vi "PrefDialog.vi"(8 "error in (no error)":errorcluster, 11 "Agilent_3458":refnum<class "Agilent_3458.lvclass">) -> (0 "error out":errorcluster, 3 "Agilent_3458":refnum<class "Agilent_3458.lvclass">)   [LabVIEW 2018, in "DigitizerPlugins.lvlib" / "Agilent_3458.lvclass"]
uses:
  Agilent_3458.lvclass
  F:/Projects/ICDAS/NistPluggableModules/Digitizer/DigitizerPlugins/DigitizerBaseClass/DigitizerBase.lvclass
  F:/Program Files (x86)/National Instruments/LabVIEW 2018/user.lib/NIST/BaseClasses/BasePlugin_class/BasePlugin.lvclass
  DigitizerBaseClass/Typedefs/Channel.ctl
  DigitizerBaseClass/Typedefs/Trigger.ctl
  DigitizerBaseClass/Typedefs/TrigSource.ctl
  DigitizerBaseClass/Typedefs/Acquisition.ctl
  DigitizerBaseClass/DigitizerBase.lvclass/DigitizerBase.ctl
  Agilent_3458.lvclass/Agilent_3458.ctl
  <userlib>/NIST/BaseClasses/BasePlugin_class/BasePlugin.lvclass/BasePlugin.ctl
  DigitizerBaseClass/Accessors/Read Acquisition.vi
  Accessors/Read Function (0_ DC Voltage).vi
  DigitizerBaseClass/Accessors/Read Channels.vi
  DigitizerBaseClass/Accessors/Read Trigger.vi
  DigitizerBaseClass/Accessors/Read Handle.vi
  <userlib>/NIST/BaseClasses/BasePlugin_class/Accessors/Read PluginIniFilePath.vi
  DigitizerBaseClass/Accessors/Write Handle.vi
  DigitizerBaseClass/Accessors/Write Channels.vi
  DigitizerBaseClass/Accessors/Write Trigger.vi
  Accessors/Write Function (0_ DC Voltage).vi
  DigitizerBaseClass/Accessors/Write Acquisition.vi
  <userlib>/NIST/BaseClasses/BasePlugin_class/Accessors/Write PluginIniFilePath.vi
  <vilib>/Utility/config.llb/NI_LVConfig.lvlib
  DigitizerPlugins.lvlib
  DigitizerBaseClass/DigitizerBase.lvclass
panel:
  in  "Handle":string
  in  "btnSaveAs":bool
  in  "btnSave":bool
  in  "btnCancel":bool
  in  "Tab Control":enum32{"Channels", "Acquisition", "Trigger"}(tab)
  in  "Channel":T1
  in  "Function (0: DC Voltage)":u16(ring) items=["DC Voltage", "AC Voltage", "AC + DC Voltage", "DC Current", "AC Current", "AC + DC Current", "2-Wire Resistance", "4-Wire Resistance", "Frequency", "Period", "Direct Sampling DC", "Direct Sampling AC", "Sub-Sampling DC", "Sub-Sampling AC"]
  in  "Acquisition":T2 {"SampleMode" items=["Real Time", "Equivalent Time"]}
  in  "Trigger":T3
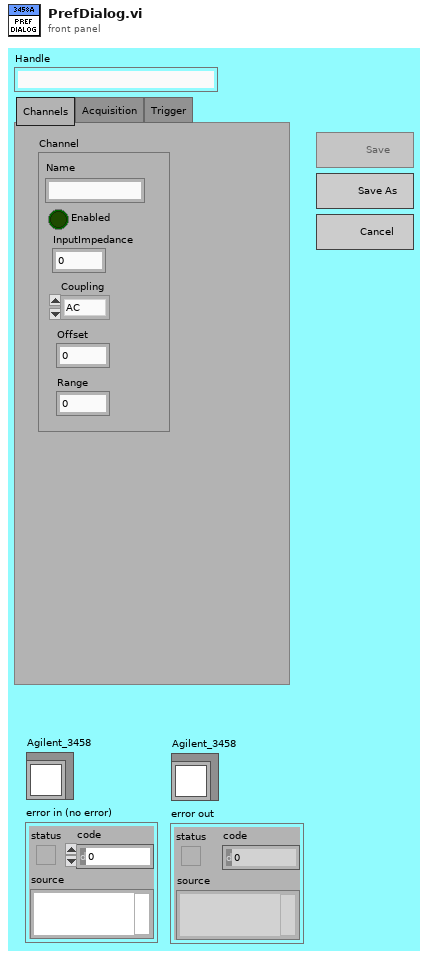
[diagram p1: front panel]
types:
  T1 = typedef "DigitizerPlugins.lvlib/DigitizerBase.lvclass/Channel.ctl" = cluster{"Name":string, "Enabled":bool, "InputImpedance":dbl, "Coupling":enum16{"AC", "DC", "Gnd"}, "Offset":dbl, "Range":dbl}
  T2 = typedef "DigitizerPlugins.lvlib/DigitizerBase.lvclass/Acquisition.ctl" = cluster{"SampleRate":dbl, "RecordSize":i32, "NumRecords":i32, "SampleMode":i32, "Timeout (ms)":i32}
  T3 = typedef "DigitizerPlugins.lvlib/DigitizerBase.lvclass/Trigger.ctl" = cluster{"Source":string, "Delay":dbl, "Holdoff":dbl, "PretriggerSamples":i32, "Sources":T4[]}
  T4 = typedef "DigitizerPlugins.lvlib/DigitizerBase.lvclass/TrigSource.ctl" = cluster{"Name":string, "Coupling":enum16{"AC", "DC", "HF Reject", "LF Reject", "Noise Reject"}, "Hysteresis":dbl, "Level":dbl, "Slope":enum16{"Positive", "Negative"}, "Type":enum16{"Edge", "Width", "Runt", "Glitch", "TV", "Window"}}
  T5 = enum32{"Invalid", "Default", "Floating", "Floating/Auto-Hide", "Modal"}
  T6 = enum8{"Enabled", "Disabled", "Disabled and Grayed Out"}
  T7 = typedef "NI_LVConfig.lvlib/Config Data RefNum.ctl" = refnum<k1>
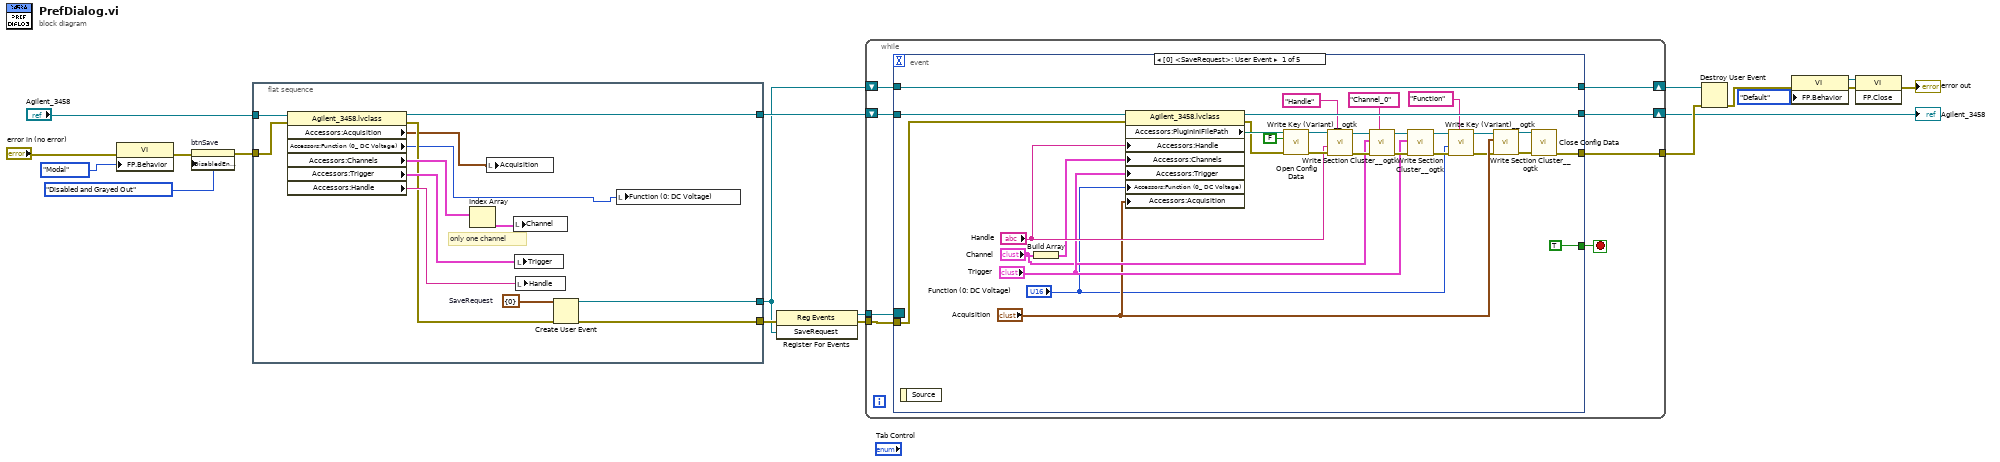
[diagram p0: block diagram]
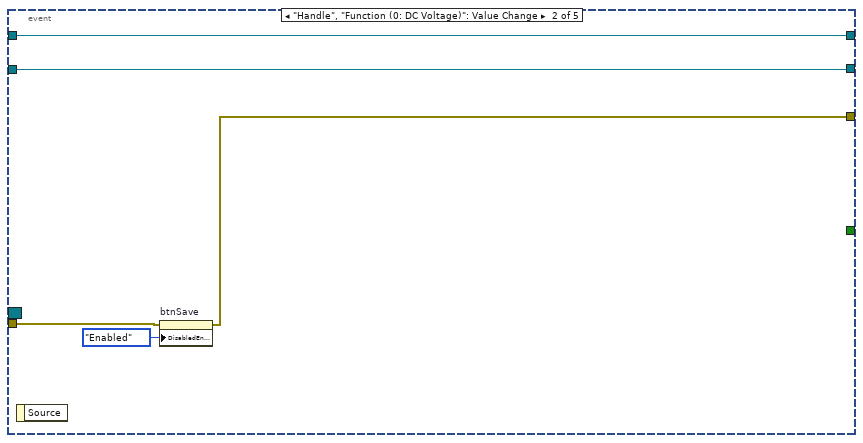
[diagram p2: hidden frame]
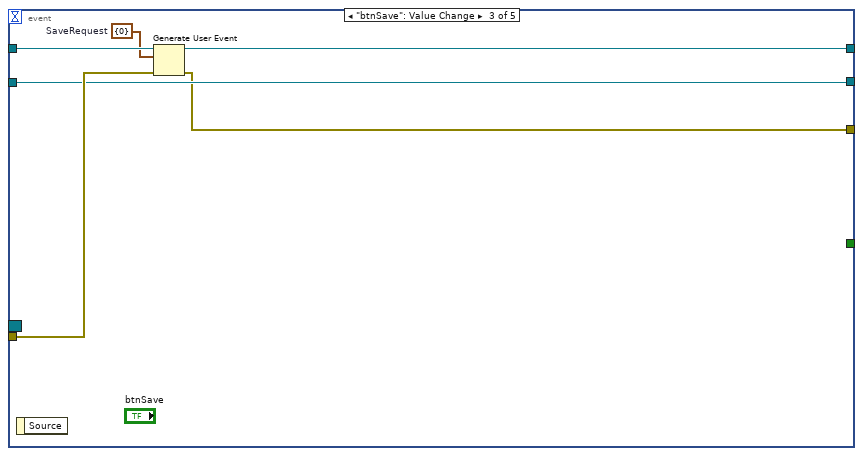
[diagram p3: hidden frame]
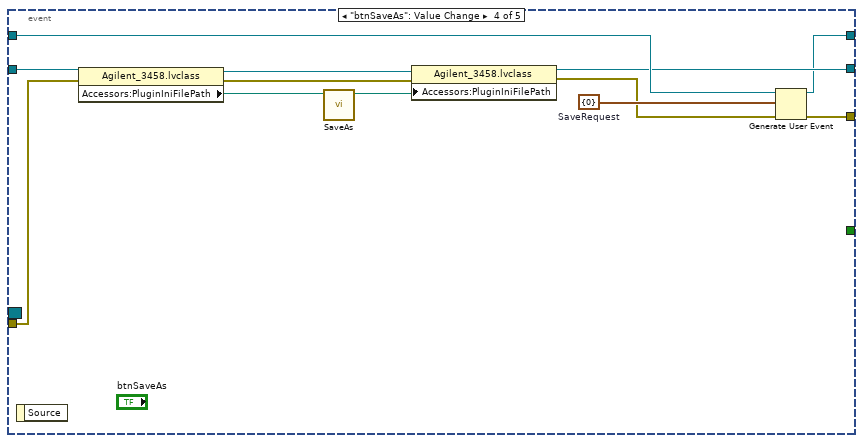
[diagram p4: hidden frame]
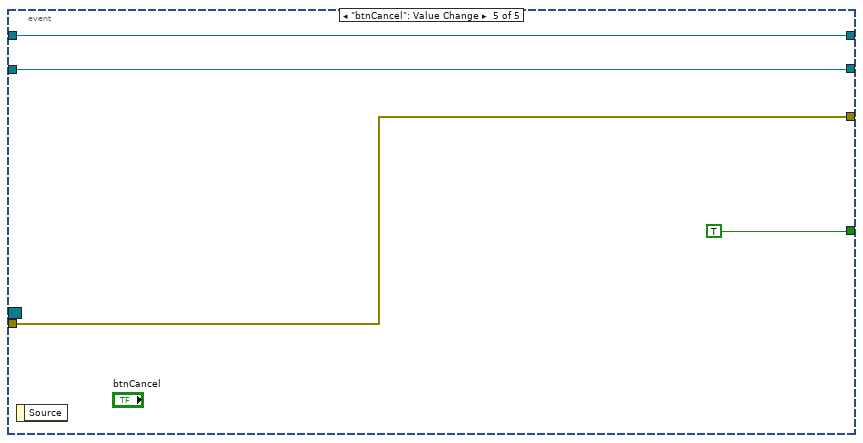
[diagram p5: hidden frame]
diagram:
  n1 = property class="VI"(error in="error in (no error)", "FP.Behavior"=T5."Modal" ("Front Panel Window:Behavior")) -> (error out=w17:errorcluster)  [unwired: 1 in, 1 out]
  n2 = property on="btnSave" class="Bool"(error in=w17, "DisabledEnum"=T6."Disabled and Grayed Out" ("Disabled")) -> (error out=w14:errorcluster)  [unwired: 1 in, 1 out]
  n3 = flat-sequence {
    tunnel: "Agilent_3458" -> [w32]
    tunnel: w14 -> [w31]
    tunnel: [w24] -> w9
    tunnel: [w23] -> w13
    tunnel: [w22] -> w10
    frame #0 {
      w25 = cluster{"num":i32} {"num"=0}  # SaveRequest
      # "only one channel"
      n4 = property class="Agilent_3458.lvclass"(reference=w32, error in=w31) -> (reference out=w22:refnum<class "Agilent_3458.lvclass">, error out=w26:errorcluster, "Accessors:Acquisition"=w20:T2, "Accessors:Function (0_ DC Voltage)"=w21:u16, "Accessors:Channels"=w30:T1[], "Accessors:Trigger"=w28:T3, "Accessors:Handle"=w27:string)
      n5 = Index Array(array=w30) -> (element=w29:T1)  [unwired: 1 in]
      n6 = local write "Acquisition"(w20) -> ()
      n7 = local write "Channel"(w29) -> ()
      n8 = local write "Trigger"(w28) -> ()
      n9 = local write "Handle"(w27) -> ()
      n10 = Create User Event(user event datatype=w25, error in=w26) -> (user event=w24:refnum<user-event>, error out=w23:errorcluster)
      n11 = local write "Function (0: DC Voltage)"(w21) -> ()
    }
  }
  n12 = register-events(error in=w13, w9) -> (reference out=w11:refnum<event-registration>, error out=w12:errorcluster)  [unwired: 1 in]
  n13 = while {
    tunnel: w12 -> [w40]
    tunnel: w11 -> [w39]
    shift-right: [w36] -> w6
    shift-left: w10 -> [w38]
    shift-right: [w34] -> w8
    shift-left: w9 -> [w35]
    tunnel: [w33] -> w7
    stop <- w37 stop-if-true
    n14 = event shown="[0] <SaveRequest>: User Event" {
      selector: w39 -> [_ _ _ _ _]
      dyn-events: _ -> [_ _ _ _ _]
      timeout: _ -> [_ _ _ _ _]
      tunnel: w40 -> [w69 w73 w79 w92 w94]
      tunnel: w38 -> [w70 w75 w78 w93 w95]
      tunnel: [TRUE _ _ _ TRUE] -> w37
      tunnel: [w55 w75 w78 w86 w95] -> w36
      tunnel: w35 -> [w54 w71 w81 w87 w96]
      tunnel: [w54 w71 w77 w82 w96] -> w34
      tunnel: [w53 w72 w76 w83 w94] -> w33
      event User Event {
        n15 = event-data() -> ()  [unwired: 1 in, 1 out]
        n16 = Build Array("Channel") -> (w60:T1[])
        n17 = property class="Agilent_3458.lvclass"(reference=w70, error in=w69, "Accessors:Handle"="Handle", "Accessors:Channels"=w60, "Accessors:Trigger"="Trigger", "Accessors:Function (0_ DC Voltage)"="Function (0: DC Voltage)", "Accessors:Acquisition"="Acquisition") -> (reference out=w55:refnum<class "Agilent_3458.lvclass">, error out=w66:errorcluster, "Accessors:PluginIniFilePath"=w68:path)
        n18 = call <vilib>:"Open Config Data.vi"("error in (no error)"=w66, "create file if necessary (T)"=FALSE, "configuration file path"=w68) -> ("error out"=w65:errorcluster, "refnum"=w64:T7)  [unwired: 6 in, 1 out]
        n19 = call <userlib>:"Write Key (Variant)__ogtk.vi"("section"="Handle", "error in (no error)"=w65, "key-value"="Handle", "refnum"=w64) -> ("error out"=w62:errorcluster, "refnum out"=w61:T7)  [unwired: 6 in]
        n20 = call <userlib>:"Write Section Cluster__ogtk.vi"("section (optional)"="Channel_0", "error in (no error)"=w62, "Section Formatted Cluster"="Channel", "refnum"=w61) -> ("error out"=w59:errorcluster, "dup refnum"=w58:T7)  [unwired: 6 in]
        n21 = call <userlib>:"Write Section Cluster__ogtk.vi"("error in (no error)"=w59, "Section Formatted Cluster"="Trigger", "refnum"=w58) -> ("error out"=w46:errorcluster, "dup refnum"=w45:T7)  [unwired: 7 in]
        n22 = call <userlib>:"Write Key (Variant)__ogtk.vi"("section"="Function", "error in (no error)"=w46, "key-value"="Function (0: DC Voltage)", "refnum"=w45) -> ("error out"=w44:errorcluster, "refnum out"=w43:T7)  [unwired: 6 in]
        n23 = call <userlib>:"Write Section Cluster__ogtk.vi"("error in (no error)"=w44, "Section Formatted Cluster"="Acquisition", "refnum"=w43) -> ("error out"=w49:errorcluster, "dup refnum"=w48:T7)  [unwired: 7 in]
        n24 = call <vilib>:"Close Config Data.vi"("error in (no error)"=w49, "refnum"=w48) -> ("error out"=w53:errorcluster)  [unwired: 8 in, 1 out]
      }
      event "Handle", "Function (0: DC Voltage)": Value Change {
        n25 = event-data() -> ()  [unwired: 1 in, 1 out]
        n26 = property on="btnSave" class="Bool"(error in=w73, "DisabledEnum"=T6."Enabled" ("Disabled")) -> (error out=w72:errorcluster)  [unwired: 1 in, 1 out]
      }
      event "btnSave": Value Change {
        w80 = cluster{"num":i32} {"num"=0}  # SaveRequest
        n27 = event-data() -> ()  [unwired: 1 in, 1 out]
        n28 = Generate User Event(user event=w81, event data cluster=w80, error in=w79) -> (user event out=w77:refnum<user-event>, error out=w76:errorcluster)  [unwired: 1 in]
      }
      event "btnSaveAs": Value Change {
        w85 = cluster{"num":i32} {"num"=0}  # SaveRequest
        n29 = event-data() -> ()  [unwired: 1 in, 1 out]
        n30 = property class="Agilent_3458.lvclass"(reference=w93, error in=w92) -> (reference out=w90:refnum<class "Agilent_3458.lvclass">, error out=w89:errorcluster, "Accessors:PluginIniFilePath"=w91:path)
        n31 = call "SaveAs.vi"("PluginIniFilePath"=w91) -> ("PluginIniFilePath"=w88:path)  [unwired: 10 in]
        n32 = property class="Agilent_3458.lvclass"(reference=w90, error in=w89, "Accessors:PluginIniFilePath"=w88) -> (reference out=w86:refnum<class "Agilent_3458.lvclass">, error out=w84:errorcluster)
        n33 = Generate User Event(user event=w87, event data cluster=w85, error in=w84) -> (user event out=w82:refnum<user-event>, error out=w83:errorcluster)  [unwired: 1 in]
      }
      event "btnCancel": Value Change {
        n34 = event-data() -> ()  [unwired: 1 in, 1 out]
      }
    }
  }
  "Agilent_3458" <- w6
  n35 = Destroy User Event(user event=w8, error in=w7) -> (error out=w5:errorcluster)
  n36 = property class="VI"(error in=w5, "FP.Behavior"=T5."Default" ("Front Panel Window:Behavior")) -> (reference out=w2:refnum<vi>, error out=w3:errorcluster)  [unwired: 1 in]
  n37 = invoke class="VI" method="FP.Close"(reference=w2, error in=w3) -> (error out=→"error out":errorcluster)  [unwired: 1 in, 2 out]
